vi "DO Module Tags.vi"(11 "DO Module Config":T6(array[cluster]) {"Settings"."Valve Settings"."D-O Settings"."Output Channel" items=["Choose a Channel"]}) -> (2 "DO Tags Array":T7[](array[typedef]), 3 "All  Numeric Tags":string[](array[string]))   [LabVIEW 2018, in "D-O Module.lvlib"]
uses:
  D-O Module Tag Names Cluster.ctl
  <vilib>/Utility/miscctls.llb/LVPoint32TypeDef.ctl
  Valve Clusters.ctl
  D-O Module Settings Cluster.ctl
  D-O Device Settings Cluster.ctl
  VICI Electronic Actuator/VICI Electronic Actuator Settings.ctl
  D-O Module.lvlib
  DIO Valve/VICI Electronic Actuator.lvlib
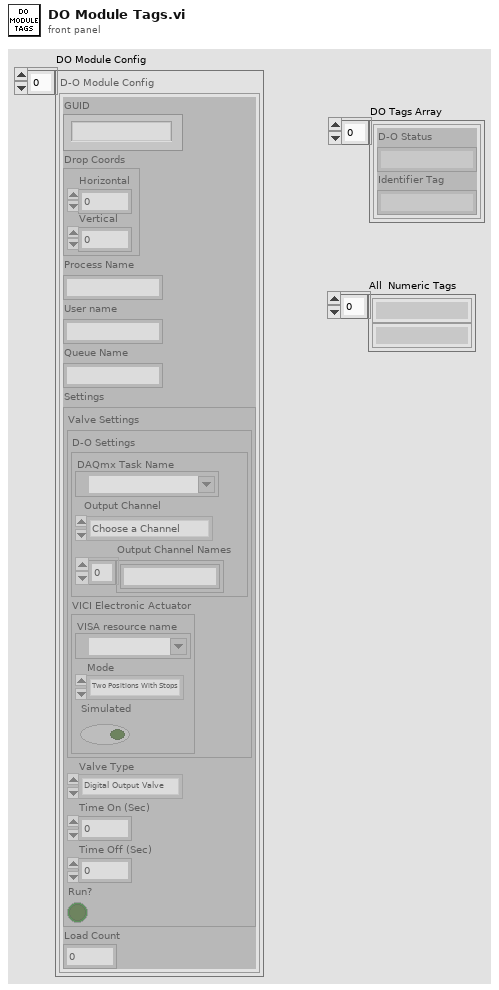
[diagram p1: front panel]
types:
  T1 = typedef "LVPoint32TypeDef.ctl" = cluster{"Horizontal":i32, "Vertical":i32}
  T2 = typedef "D-O Module.lvlib/Valve Clusters.ctl" = cluster{"Valve Settings":T3, "Valve Type":enum16{"Default", "Digital Output Valve", "VICI Electronic Actuator"}, "Time On (Sec)":dbl, "Time Off (Sec)":dbl, "Run?":bool}
  T3 = typedef "D-O Module.lvlib/D-O Module Settings Cluster.ctl" = cluster{"D-O Settings":T4, "VICI Electronic Actuator":T5}
  T4 = typedef "D-O Module.lvlib/D-O Device Settings Cluster.ctl" = cluster{"DAQmx Task Name":refnum<k21>, "Output Channel":u16, "Output Channel Names":string[]}
  T5 = typedef "VICI Electronic Actuator.lvlib/VICI Electronic Actuator Settings.ctl" = cluster{"VISA resource name":refnum<visa-resource-name>, "Mode":enum16{"Two Positions With Stops", "Two Positions Without Stops", "Mutiposition"}, "Simulated":bool}
  T6 = cluster{"GUID":string, "Drop Coords":T1, "Process Name":string, "User name":string, "Queue Name":string, "Settings":T2, "Load Count":i32}[]
  T7 = typedef "D-O Module.lvlib/D-O Module Tag Names Cluster.ctl" = cluster{"D-O Status":string, "Identifier Tag":string}
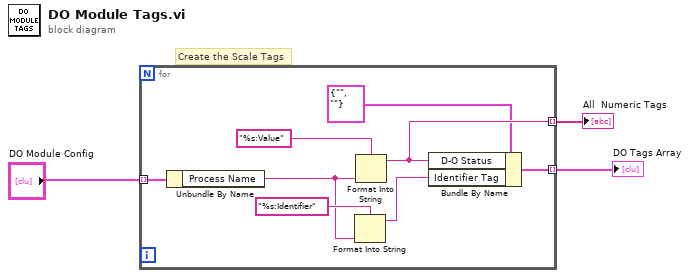
[diagram p0: block diagram]
diagram:
  # "Create the Scale Tags"
  n1 = for {
    tunnel: "DO Module Config" -> [w8] mode=indexing
    tunnel: [w9] -> w3 mode=indexing
    tunnel: [w10] -> w2 mode=indexing
    n2 = Unbundle By Name(w8) -> ("Process Name"=w6:string)
    n3 = Format Into String(format string="%s:Identifier", w6) -> (resulting string=w5:string)  [unwired: 2 in, 1 out]
    n4 = Format Into String(format string="%s:Value", w6) -> (resulting string=w10:string)  [unwired: 2 in, 1 out]
    n5 = Bundle By Name(cluster=T7 {"D-O Status"="", "Identifier Tag"=""} ("D-O Module Tag Names"), "D-O Status"=w10, "Identifier Tag"=w5) -> (w9:T7)
  }
  "DO Tags Array" <- w3
  "All  Numeric Tags" <- w2
